vi "E-S WITHOUT START SESSION.vi"(4 "ID ESPERADO STRING":string, 5 "string":string, 6 "ID":string, 7 "Read":refnum<k21>, 8 "Write":refnum<k21>) -> (2 "Data String":string, 3 "ID String":string)   [LabVIEW 2022 SP3]
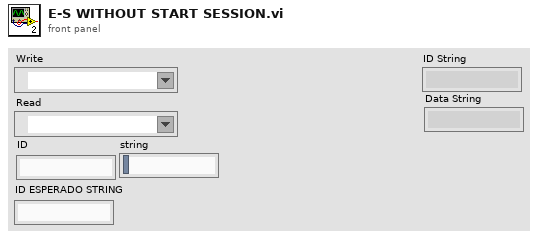
[diagram p1: front panel]
types:
  T1 = typedef "XNET Frame CAN.ctl" = cluster{"timestamp":timestamp, "payload":u8[], "identifier":u32, "type":T2, "extended?":bool, "echo?":bool}
  T2 = typedef "XNET Frame Type CAN.ctl" = u8
  T3 = cluster{"data[0]":T1, "data[1]":T1, "data[2]":T1, "data[3]":T1, "data[4]":T1, "data[5]":T1, "data[6]":T1, "data[7]":T1, "data[8]":T1}
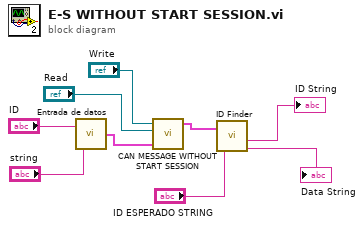
[diagram p0: block diagram]
diagram:
  n1 = call "Entrada de datos.vi"("string"="string", "ID"="ID") -> ("CAN frame"=w9:T1)
  n2 = call "CAN MESSAGE WITHOUT START SESSION.vi"("CAN frame"=w9, "Read"="Read", "Write"="Write") -> ("cluster"=w4:T3)  [unwired: 1 in, 1 out]
  n3 = call "ID Finder.vi"("cluster"=w4, "ID ESPERADO STRING"="ID ESPERADO STRING") -> ("ID String"=→"ID String":string, "Data String"=→"Data String":string)  [unwired: 4 out]
